vi "Get Owning Path Default Value.vi"(0 "SG Path Group in":refnum<class "SG Path Group.lvclass">, 11 "error in":errorcluster) -> (4 "SG Path Group out":refnum<class "SG Path Group.lvclass">, 6 "Path":refnum<class "Path.lvclass">, 15 "error out":errorcluster)   [LabVIEW 2023, in "RFFixtureCharact.RMM.lvlib" / "SG Path Group.lvclass"]
uses:
  SG Path Group.lvclass
  Common/Base Classes/Path/Path.lvclass
  Public/Base Classes/Scalar/SG Path/SG Path.lvclass
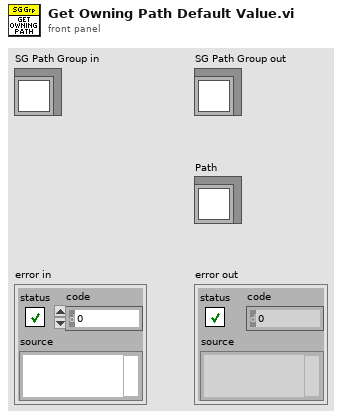
[diagram p1: front panel]
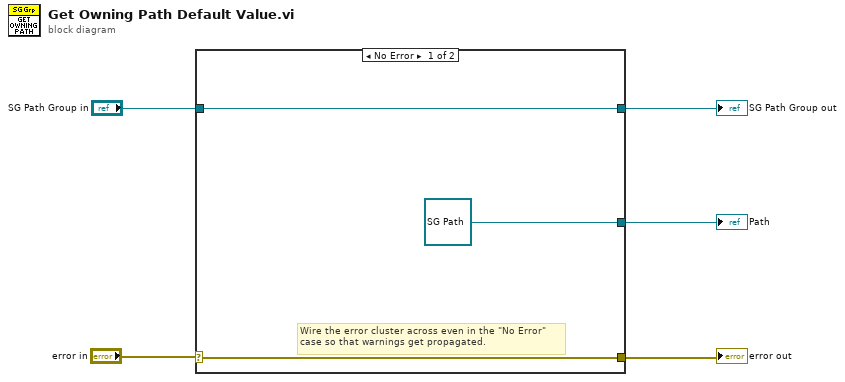
[diagram p0: block diagram]
diagram:
  n1 = case shown="No Error" "error in" {
    selector: "error in" -> [w7 w10]
    tunnel: [w7 w10] -> w5
    tunnel: [w8 w9] -> w2
    tunnel: "SG Path Group in" -> [w8 w9]
    tunnel: [refnum<class "SG Path.lvclass"> refnum ("RFFixtureCharact.Public.lvlib:SG Path.lvclass") _] -> w3
    frame No Error {
      # "Wire the error cluster across even in the \"No Error\"\ncase so that warnings get propagated."
    }
    frame Error {
    }
  }
  "error out" <- w5
  "SG Path Group out" <- w2
  "Path" <- w3
